vi "POLL BIAS (MTDC).vi"(8 "error in (no error)":errorcluster, 9 "Port number (3364)":u32=3364, 10 "ScanQ in":refnum<queue>, 11 "SweepQ in":refnum<queue>) -> (0 "error out":errorcluster, 2 "ScanQ out":refnum<queue>, 3 "SweepQ out":refnum<queue>)   [LabVIEW 2025]
uses:
  <userlib>/Nanonis Prog Interface V5e/Nanonis Prog Interface.lvlib
  STM-Auto-Project/QMH CTLS/Scan_Params (QMH).ctl
  STM-Auto-Project/QMH CTLS/Sweeper.ctl
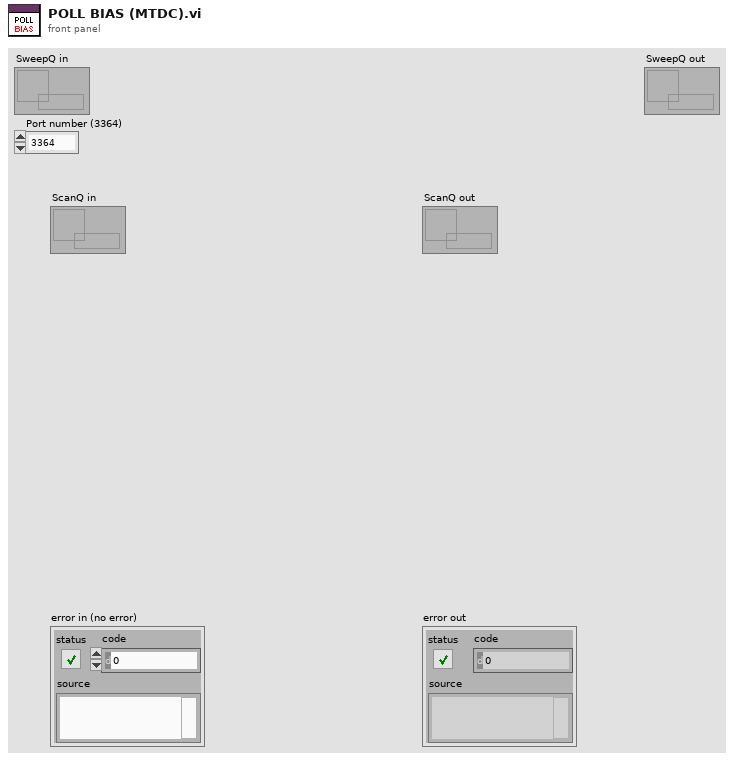
[diagram p1: front panel]
types:
  T1 = enum16{"1. BIAS", "2. INIT_SCAN", "3. SCAN_IDLE", "4. INTER_SCAN", "5. NEW_COORDS_&_FRAME", "6. FINAL_SCAN", "7. POLL BIAS ", "8. STOP"}
  T2 = typedef "Scan_Params (QMH).ctl" = cluster{"Setpoint (I)":dbl[], "Bias (V)":dbl[], "Number of scans":u8, "Port number (3364)":u32, "Avoid zero threshold (V)":dbl, "Current State":enum16{"1. BIAS", "2. INIT_SCAN", "3. SCAN_IDLE", "4. INTER_SCAN", "5. NEW_COORDS_&_FRAME", "6. FINAL_SCAN", "7. POLL BIAS ", "8. STOP"}}
  T3 = enum16{"NO CHANGE", "SET TEMP & FIELD", "SWEEP IDLE", "NEXT TEMP & FIELD", "SWEEP DONE"}
  T4 = typedef "Sweeper.ctl" = cluster{"Temps(K)":dbl[], "Fields(T)":dbl[], "Sweep States":enum16{"NO CHANGE", "SET TEMP & FIELD", "SWEEP IDLE", "NEXT TEMP & FIELD", "SWEEP DONE"}}
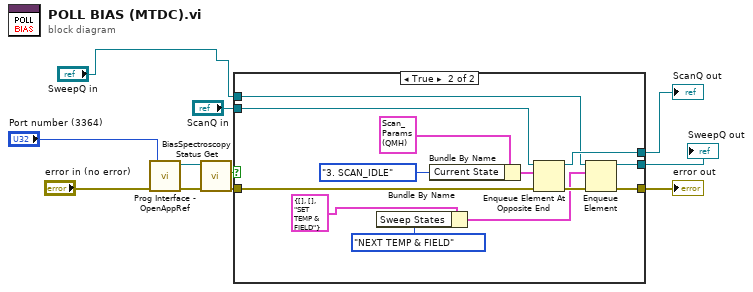
[diagram p0: block diagram]
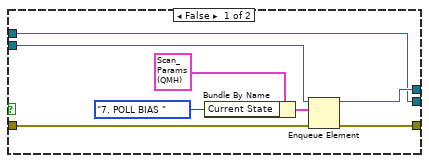
[diagram p2: hidden frame]
diagram:
  n1 = call <userlib>:"Prog Interface - OpenAppRef.vi"("Error in (no error)"="error in (no error)", "Port number (3364)"="Port number (3364)") -> ("Error out"=w6:errorcluster, "Application reference"=w5:refnum<vi>)  [unwired: 4 in]
  n2 = call <userlib>:"BiasSpectroscopy Status Get.vi"("Error in (no error)"=w6, "Application ref in"=w5) -> ("Error out"=w11:errorcluster, "Running?"=w7:bool)  [unwired: 5 in, 1 out]
  n3 = case shown="True" w7 {
    tunnel: "ScanQ in" -> [w19 w32]
    tunnel: [w15 w28] -> w9
    tunnel: "SweepQ in" -> [w12 w27]
    tunnel: [w12 w26] -> w3
    tunnel: [w13 w24] -> w10
    tunnel: w11 -> [w14 w23]
    frame False {
      n4 = Bundle By Name(cluster=T2 {"Setpoint (I)"=[], "Bias (V)"=[], "Number of scans"=1, "Port number (3364)"=3364, "Avoid zero threshold (V)"=0.004999999888241291, "Current State"=enum."1. BIAS"} ("element"), "Current State"=T1."7. POLL BIAS ") -> (w16:T2)
      n5 = Enqueue Element(queue=w19, element=w16, error in (no error)=w14) -> (queue out=w15:refnum<queue>, error out=w13:errorcluster)  [unwired: 1 in, 1 out]
    }
    frame True {
      n6 = Bundle By Name(cluster=T4 {"Temps(K)"=[], "Fields(T)"=[], "Sweep States"=enum."SET TEMP & FIELD"} ("Temp and Field Range"), "Sweep States"=T3."NEXT TEMP & FIELD") -> (w21:T4)
      n7 = Bundle By Name(cluster=T2 {"Setpoint (I)"=[], "Bias (V)"=[], "Number of scans"=1, "Port number (3364)"=3364, "Avoid zero threshold (V)"=0.004999999888241291, "Current State"=enum."1. BIAS"} ("element"), "Current State"=T1."3. SCAN_IDLE") -> (w29:T2)
      n8 = Enqueue Element At Opposite End(queue=w32, element=w29, error in (no error)=w23) -> (queue out=w28:refnum<queue>, error out=w25:errorcluster)  [unwired: 1 in, 1 out]
      n9 = Enqueue Element(queue=w27, element=w21, error in (no error)=w25) -> (queue out=w26:refnum<queue>, error out=w24:errorcluster)  [unwired: 1 in, 1 out]
    }
  }
  "error out" <- w10
  "ScanQ out" <- w9
  "SweepQ out" <- w3
